vi "LaserOFF.vi"(8 "error in":errorcluster, 10 "ON/OFF":bool, 11 "VISA resource name in":refnum<visa-resource-name>) -> (0 "error out":errorcluster, 3 "VISA resource name out":refnum<visa-resource-name>)   [LabVIEW 2014]
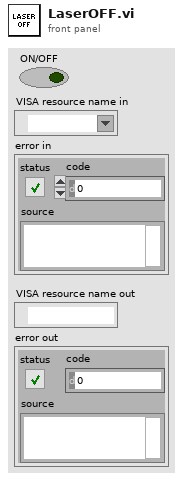
[diagram p1: front panel]
types:
  T1 = cluster{"D0 latched power setting":bool, "D1 latched power setting":bool, "D2 latched power setting":bool, "D3 latched power setting":bool, "D4 latched power setting":bool, "D5 latched power setting":bool, "D6 latched power setting":bool, "D7 latched power setting":bool, "D0 power setting":bool, "D1 power setting":bool, "D2 power setting":bool, "D3 power setting":bool, "D4 power setting":bool, "D5 power setting":bool, "D6 power setting":bool, "D7 power setting":bool, "Latch":bool, "Auxiliary Emission OFF":bool, "Emission Modulation":bool, "Guide laser control":bool, "External Synchronization Input":bool, "Emission enable":bool, "Serial Input":bool, "Serial Clock":bool, "State0":bool, "State1":bool, "State2":bool, "Serial Output":bool, "Serial Enable":bool, "Reserved [29]":bool, "Reserved [30]":bool, "Reserved [31]":bool}
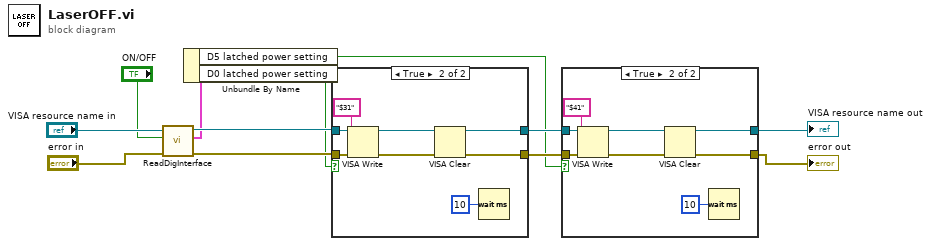
[diagram p0: block diagram]
diagram:
  n1 = call "ReadDigInterface.vi"("error in"="error in", "ON/OFF"="ON/OFF", "VISA resource name in"="VISA resource name in") -> ("error out"=w11:errorcluster, "Extend Device Status"=w7:T1, "VISA resource name out"=w12:refnum<visa-resource-name>)  [unwired: 5 in]
  n2 = Unbundle By Name(w7) -> ("D5 latched power setting"=w2:bool, "D0 latched power setting"=w1:bool)
  n3 = case shown="True" w1 {
    tunnel: w12 -> [w14 w22]
    tunnel: w11 -> [w13 w21]
    tunnel: [w14 w19] -> w6
    tunnel: [w13 w18] -> w5
    frame False {
    }
    frame True {
      n4 = VISA Write(VISA resource name=w22, write buffer="$31", error in (no error)=w21) -> (VISA resource name out=w16:refnum<visa-resource-name>, error out=w15:errorcluster)  [unwired: 1 out]
      n5 = VISA Clear(VISA resource name=w16, error in (no error)=w15) -> (VISA resource name out=w19:refnum<visa-resource-name>, error out=w18:errorcluster)
      n6 = Wait (ms)(milliseconds to wait=u32 10) -> ()  [unwired: 1 out]
    }
  }
  n7 = case shown="True" w2 {
    tunnel: w6 -> [w24 w32]
    tunnel: w5 -> [w23 w31]
    tunnel: [w24 w29] -> w4
    tunnel: [w23 w28] -> w3
    frame False {
    }
    frame True {
      n8 = VISA Write(VISA resource name=w32, write buffer="$41", error in (no error)=w31) -> (VISA resource name out=w26:refnum<visa-resource-name>, error out=w25:errorcluster)  [unwired: 1 out]
      n9 = VISA Clear(VISA resource name=w26, error in (no error)=w25) -> (VISA resource name out=w29:refnum<visa-resource-name>, error out=w28:errorcluster)
      n10 = Wait (ms)(milliseconds to wait=u32 10) -> ()  [unwired: 1 out]
    }
  }
  "VISA resource name out" <- w4
  "error out" <- w3
